vi "Cluster with arr of clusters to JSON.vi"() -> ()   [LabVIEW 2018]
panel:
  in  "str_arg":string
  in  "fun_name":string
  out "JSON string":string
  out "error out":errorcluster
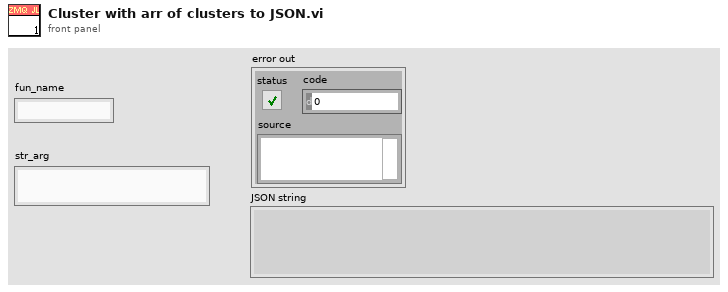
[diagram p1: front panel]
types:
  T1 = cluster{"clarray":cluster{"fun_name":string, "str_arg":string, "Byte_array":u8[]}[], "soosooo":string}
  T2 = cluster{"fun_name":string, "str_arg":string, "Byte_array":u8[]}
  T3 = cluster{"fun_name":string, "str_arg":string, "Byte_array":u8[]}[]
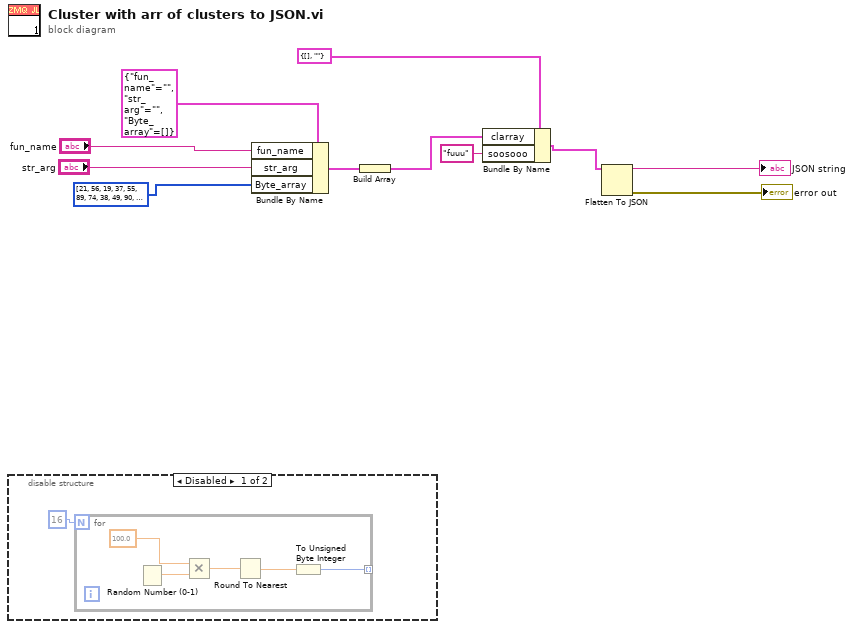
[diagram p0: block diagram]
diagram:
  n1 = disable-structure shown="Disabled" {
    frame Disabled {
      n2 = for {
        N: 16 -> [_]
        tunnel: [w13] -> _ mode=indexing
        n3 = Random Number (0-1)() -> (number: 0 to 1=w17:dbl)
        n4 = Multiply(x=100.0, y=w17) -> (x*y=w16:dbl)
        n5 = Round To Nearest(number=w16) -> (nearest integer value=w14:dbl)
        n6 = To Unsigned Byte Integer(number=w14) -> (unsigned 8bit integer=w13:u8)
      }
    }
    frame Enabled {
    }
  }
  n7 = Bundle By Name(cluster=T2 {"fun_name"="", "str_arg"="", "Byte_array"=[]} ("fun_cluster"), "fun_name"="fun_name", "str_arg"="str_arg", "Byte_array"=u8[] [21, 56, 19, 37, 55, 89, 74, 38, 49, 90, 2, 10, 96, 88, 14, 76] ("Array")) -> (w8:T2)
  n8 = Build Array(w8) -> (w3:T3)
  n9 = Bundle By Name(cluster=T1 {"clarray"=[], "soosooo"=""}, "clarray"=w3, "soosooo"="fuuu") -> (w2:T1)
  n10 = Flatten To JSON(anything=w2) -> (JSON string=→"JSON string":string, 11:→"error out":errorcluster)  [unwired: 2 in]
